vi "Write Element of Scan Engine Channels.vi"(8 "error in (no error)":errorcluster, 9 "Line":T1, 10 "index":i32, 11 "Scan Engine configuration1 in":refnum<class "Scan Engine configuration.lvclass">) -> (0 "error out":errorcluster, 3 "Scan Engine configuration1 out":refnum<class "Scan Engine configuration.lvclass">)   [LabVIEW 2015, in "Scan Engine configuration.lvclass"]
uses:
  Scan Engine configuration.lvclass
  Line.ctl
  <vilib>/NI/Tag Bus Module Framework/channel/TBM channel.lvclass
  Scan Engine configuration.lvclass/Scan Engine configuration.ctl
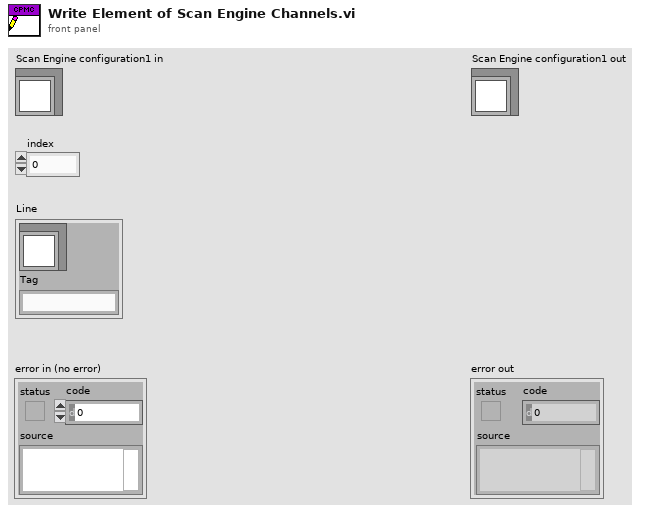
[diagram p1: front panel]
types:
  T1 = typedef "Scan Engine configuration.lvclass/Line.ctl" = cluster{"channel":refnum<class "TBM channel.lvclass">, "Tag":string}
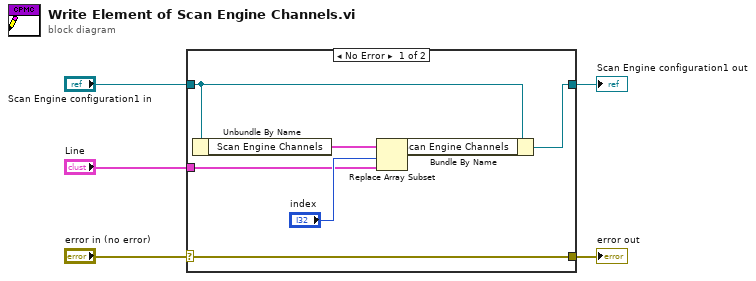
[diagram p0: block diagram]
diagram:
  n1 = case shown="No Error" "error in (no error)" {
    selector: "error in (no error)" -> [w12 w13]
    tunnel: [w12 w13] -> w4
    tunnel: [w11 w14] -> w2
    tunnel: "Scan Engine configuration1 in" -> [w10 w14]
    tunnel: "Line" -> [w6 _]
    frame No Error {
      n2 = Unbundle By Name(w10) -> ("Scan Engine Channels"=w9:T1[])
      n3 = Replace Array Subset(array=w9, new element=w6, index="index") -> (w8:T1[])
      n4 = Bundle By Name(cluster=w10, "Scan Engine Channels"=w8) -> (w11:refnum<class "Scan Engine configuration.lvclass">)
    }
    frame Error {
    }
  }
  "error out" <- w4
  "Scan Engine configuration1 out" <- w2
